vi "Update OD.vi"(9 "Action":T1, 10 "Direction":T2, 11 "Class":refnum<class "Pinwheel.lvclass">) -> (3 "Class":refnum<class "Pinwheel.lvclass">)   [LabVIEW 2020, in "Pinwheel.lvclass"]
uses:
  Pinwheel.lvclass
  Type Defs/Direction Enum.ctl
  Type Defs/Action Enum.ctl
  Pinwheel.lvclass/Pinwheel.ctl
  Type Defs/SB Type Defs.lvlib
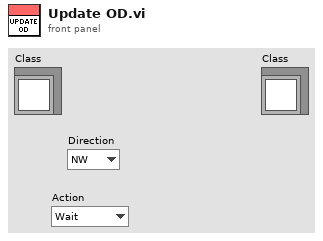
[diagram p1: front panel]
types:
  T1 = typedef "SB Type Defs.lvlib/Action Enum.ctl" = enum16{"Wait", "Move", "Attack", "Replicate"}
  T2 = typedef "SB Type Defs.lvlib/Direction Enum.ctl" = enum16{"NW", "N", "NE", "E", "SE", "S", "SW", "W"}
  T3 = typedef "Pinwheel.lvclass/DVR Cluster.ctl" = cluster{"N":i32, "E":i32, "S":i32, "W":i32, "OD":T2, "NR":i32, "ER":i32, "SR":i32, "WR":i32, "NE":i32, "EE":i32, "SE":i32, "WE":i32, "Team":i32}
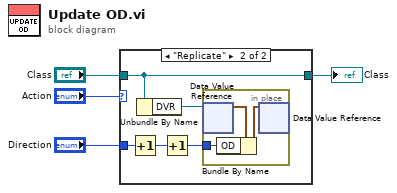
[diagram p0: block diagram]
diagram:
  n1 = case shown="\"Replicate\"" "Action" {
    tunnel: [w5 w8] -> w3
    tunnel: "Class" -> [w5 w8]
    tunnel: "Direction" -> [_ w10]
    frame Default {
    }
    frame "Replicate" {
      n2 = Increment(x=w10) -> (x+1=w9:T2)
      n3 = Unbundle By Name(w8) -> ("DVR"=w7:refnum<data-value>)
      n4 = Increment(x=w9) -> (x+1=w6:T2)
      n5 = in-place {
        in-place-border: w6 -> [w11]
        n6 = in-place-dvr #1(w7) -> (w13:T3)  [unwired: 1 out]
        n7 = Bundle By Name(cluster=w13, "OD"=w11) -> (w12:T3)
        n8 = in-place-dvr #1(w12) -> ()  [unwired: 2 out]
      }
    }
  }
  "Class" <- w3
